vi "Acquire Teardown.vi"(8 "error in (no error)":errorcluster, 11 "Top Level in":refnum<class "Top Level.lvclass">) -> (0 "error out":errorcluster, 3 "Top Level out":refnum<class "Top Level.lvclass">)   [LabVIEW 2021, in "Top Level.lvlib" / "Top Level.lvclass"]
uses:
  Top Level.lvclass
  Top Level.lvclass/Top Level.ctl
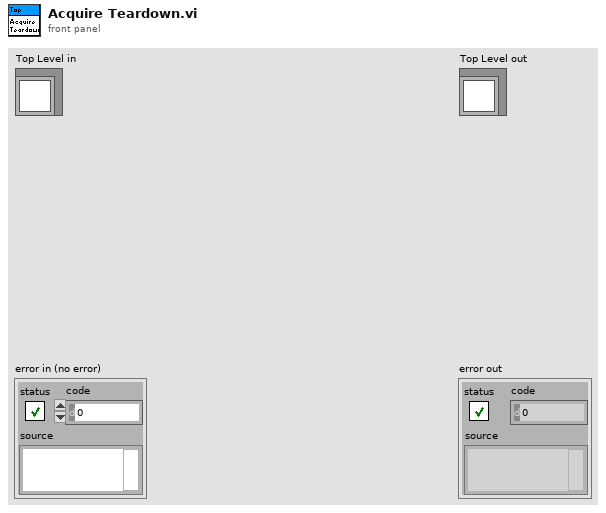
[diagram p1: front panel]
types:
  T1 = enum8{"Enabled", "Disabled", "Disabled and Grayed Out"}
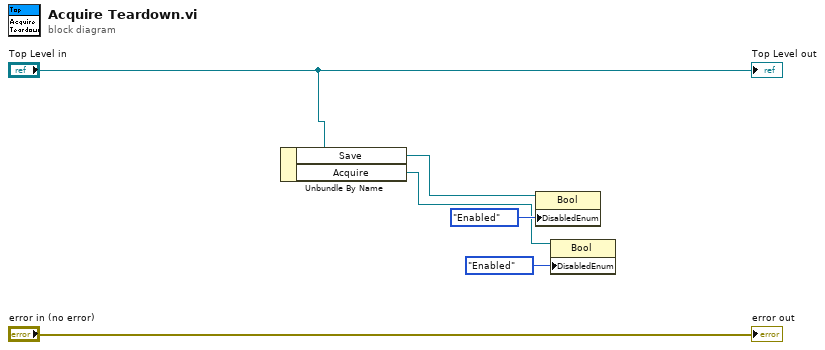
[diagram p0: block diagram]
diagram:
  n1 = Unbundle By Name("Top Level in") -> ("Save"=w5:refnum<vi>, "Acquire"=w2:refnum<vi>)
  n2 = property class="Bool"(reference=w5, "DisabledEnum"=T1."Enabled" ("Disabled")) -> ()  [unwired: 1 in, 2 out]
  n3 = property class="Bool"(reference=w2, "DisabledEnum"=T1."Enabled" ("Disabled")) -> ()  [unwired: 1 in, 2 out]
  "error out" <- "error in (no error)"
  "Top Level out" <- "Top Level in"
